vi "Try Match Response.vi"(8 "error in":errorcluster, 10 "ICAN CC Frame":refnum<class "ICAN CC Frame.lvclass">, 11 "Block Upload End Transfer in":refnum<class "Block Upload End Transfer.lvclass">) -> (0 "error out":errorcluster, 1 "SDO Result":T1={"Success"=FALSE, "SDO abort code"={"Null"=TRUE, "Value"=84082688}, "Data"={"Null"=TRUE, "Data"=[]}} {"SDO abort code"."Value" items=["Toggle bit not allowed"=84082688, "SDO protocol timed out"=84148224, "Client/server command specifier not valid or unknown"=84148225, "Invalid block size (block mode only)"=84148226, "Invalid sequence number (block mode only)"=84148227, "CRC error (block mode only)"=84148228, "Out of memory"=84148229, "Attempt to read a write only object"=100728833, "Attempt to write a read only object"=100728834, "Object does not exist in the object dictionary"=100794368, "Object cannot be mapped to the PDO"=100925505, "The number and length of the objects to be mapped would exceed PDO length"=100925506, "General parameter incompatibility reason"=100925507, "General internal incompatibility in the device"=100925511, "Access failed due to an hardware error"=101056512, "Data type does not match, length of service parameter does not match"=101122064, "Data type does not match, length of service parameter too high"=101122066, "Data type does not match, length of service parameter too low"=101122067, "Sub-index does not exist"=101253137, "Invalid value for parameter (download only)"=101253168, "Value of parameter written too high (download only)"=101253169, "Value of parameter written too low (download only)"=101253170, "Maximum value is less than minimum value"=101253174, "Resource not available: SDO connection"=101318691, "General error"=134217728, "Data cannot be transferred or stored to the application"=134217760, "Data cannot be transferred or stored to the application because of local control"=134217761, "Data cannot be transferred or stored to the application because of the present device stable"=134217762, "Object dictionary dynamic generation fails or no object dictionary is present (e.g. object dictionary is generated from file and generation fails because of an file error)"=134217763, "No data available"=134217764]; "Data"."Data" format="%02x"}, 2 "Match":bool, 3 "SDO Transfer out":refnum<class "SDO Transfer.lvclass">)   [LabVIEW 2020, in "CANopen.lvlib" / "SDO Manager.lvlib" / "Block Upload End Transfer.lvclass"]
uses:
  Block Upload End Transfer.lvclass
  HAL/Source/Interfaces/ICAN CC Frame/ICAN CC Frame.lvclass
  Block Upload End Transfer.lvclass/Block Upload End Transfer.ctl
  D:/git/CANopen-LabVIEW/source/SDO Manager/SDO Manager/SDO Transfer/SDO Transfer.lvclass
  D:/git/CANopen-LabVIEW/source/SDO Manager/SDO Manager/Block Upload End Transfer/Block Upload End Transfer.lvclass
  SDO Transfer/SDO Transfer.lvclass
  CANopen Message/CANopen Message.lvclass
  SDO Transfer/SDO abort code.ctl
  Typedefs/SDO Result.ctl
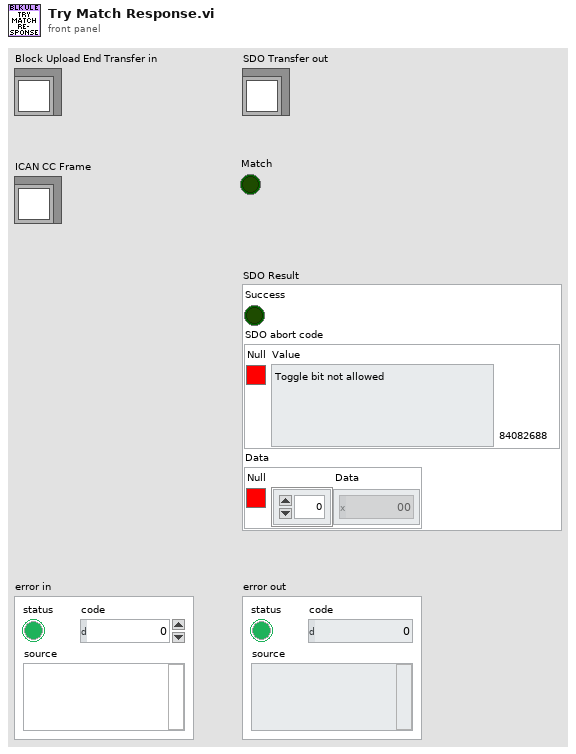
[diagram p1: front panel]
types:
  T1 = typedef "CANopen.lvlib/SDO Manager.lvlib/SDO Transfer.lvclass/SDO Result.ctl" = cluster{"Success":bool, "SDO abort code":cluster{"Null":bool, "Value":T2}, "Data":cluster{"Null":bool, "Data":u8[]}}
  T2 = typedef "CANopen.lvlib/SDO Manager.lvlib/SDO Transfer.lvclass/SDO abort code.ctl" = u32
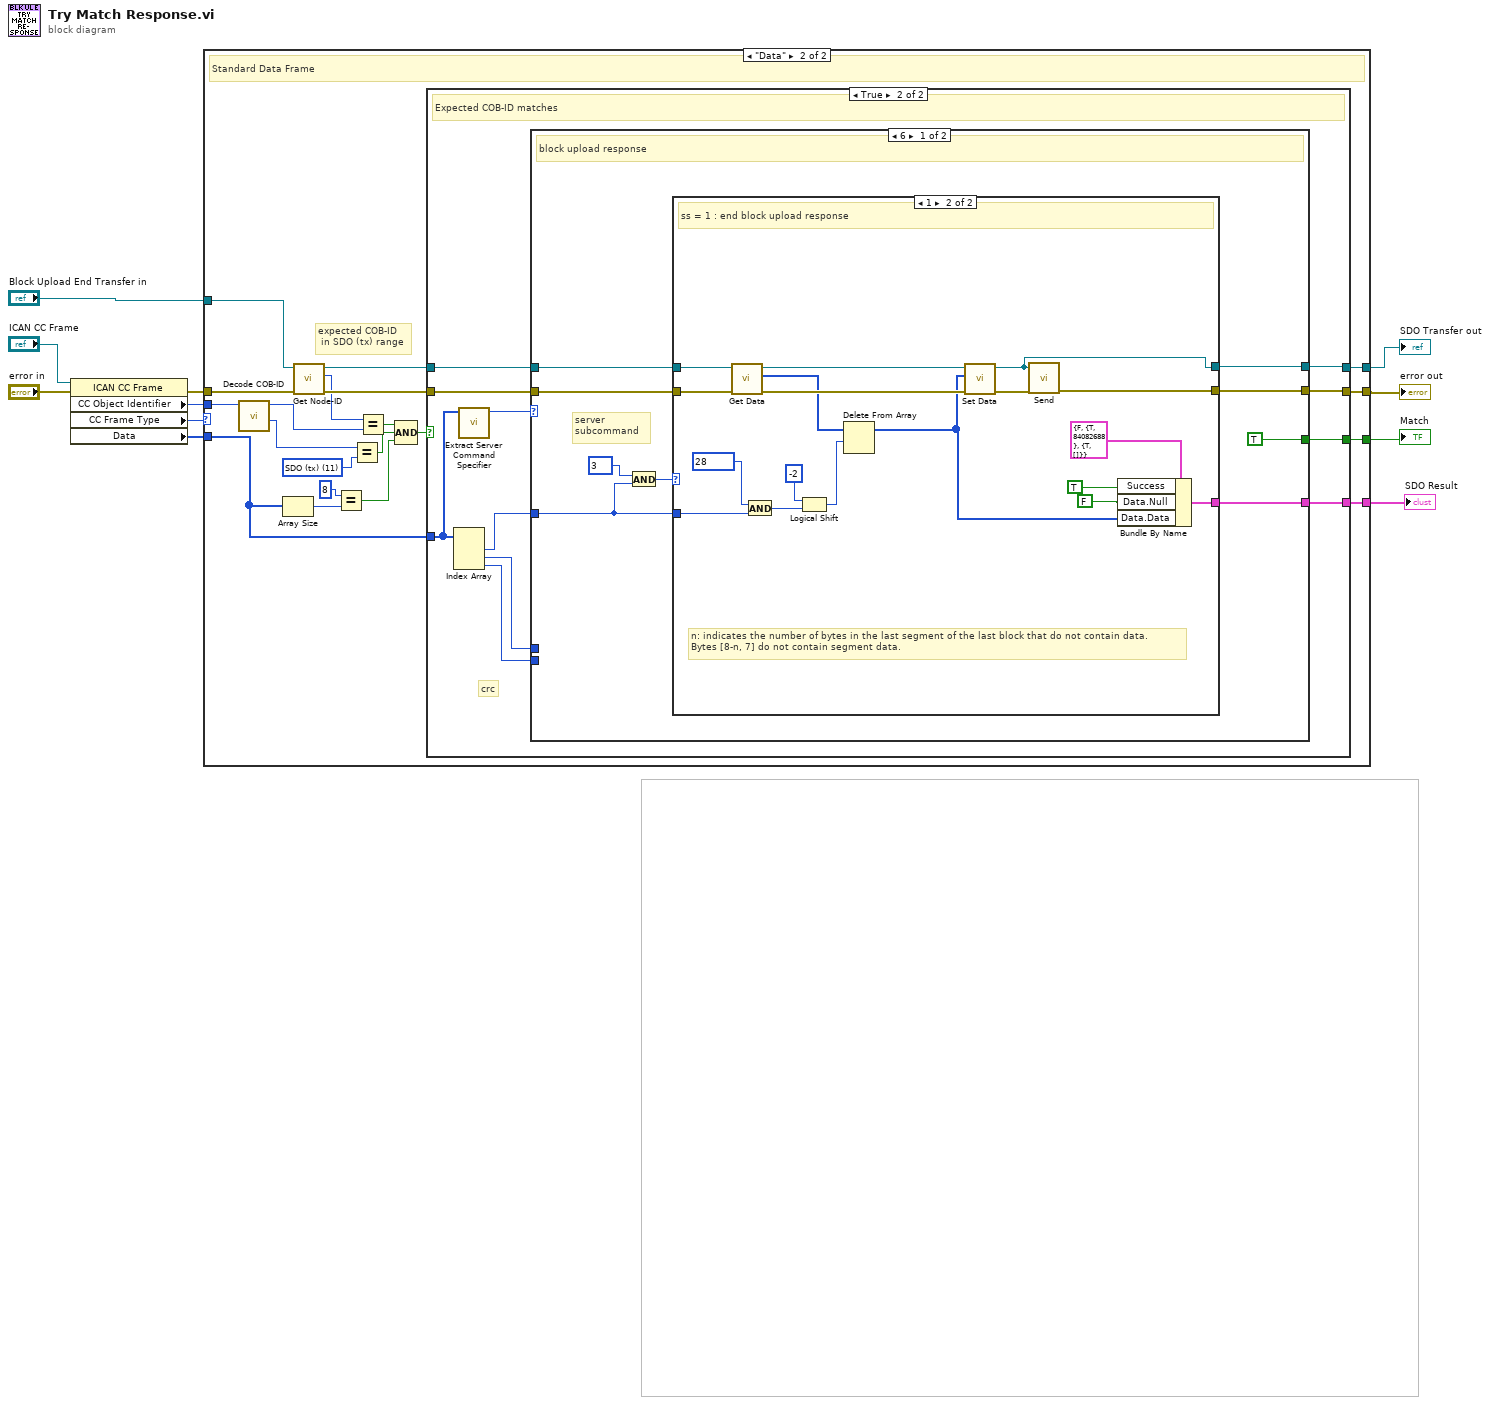
[diagram p0: block diagram]
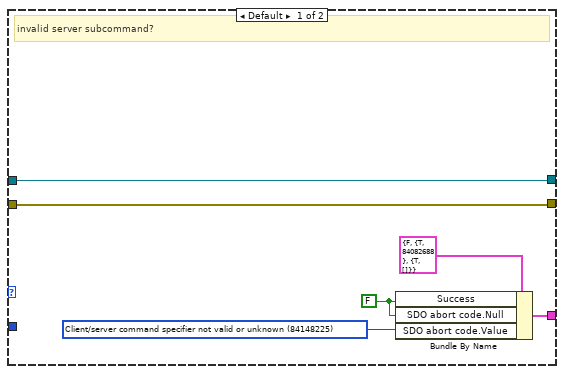
[diagram p4: hidden frame]
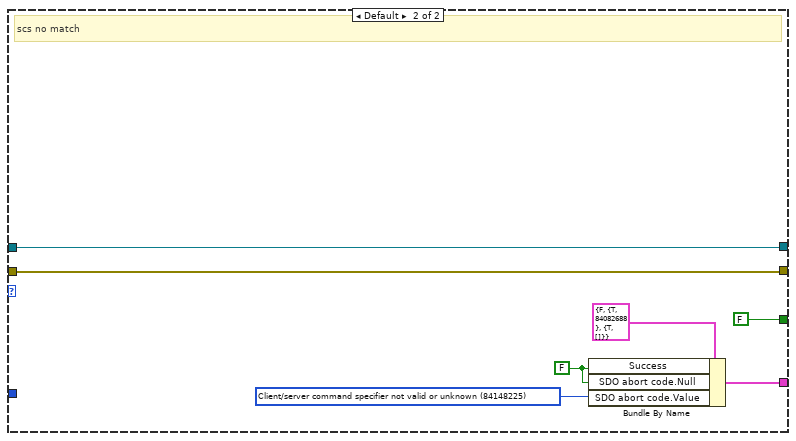
[diagram p5: hidden frame]
diagram:
  n1 = property class="ICAN CC Frame"(reference="ICAN CC Frame", error in="error in") -> (error out=w11:errorcluster, "CC Object Identifier"=w10:u32, "CC Frame Type"=w8:enum8{"Data", "Remote", "Error", "Overload"}, "Data"=w9:u8[])  [unwired: 1 out]
  n2 = case shown="\"Data\"" w8 {
    tunnel: w11 -> [w13 w33]
    tunnel: "Block Upload End Transfer in" -> [w12 w32]
    tunnel: [w12 w29] -> w5
    tunnel: [w13 w28] -> w7
    tunnel: [_ w27] -> w6
    tunnel: w10 -> [_ w26]
    tunnel: w9 -> [_ w15]
    tunnel: [_ w14] -> w1
    frame Default {
      # "Wrong Frame Type"
    }
    frame "Data" {
      w23 = u8 11 items=["NMT"=0, "EMCY/SYNC"=1, "TIME"=2, "PDO1 (tx)"=3, "PDO1 (rx)"=4, "PDO2 (tx)"=5, "PDO2 (rx)"=6, "PDO3 (tx)"=7, "PDO3 (rx)"=8, "PDO4 (tx)"=9, "PDO4 (rx)"=10, "SDO (tx)"=11, "SDO (rx)"=12, "NMT error control"=14] ("Function Code")
      # "expected COB-ID\n in SDO (tx) range"
      # "Standard Data Frame"
      n3 = call "Decode COB-ID.vi"("COD-ID"=w26) -> ("Function Code"=w22:u8, "Node-ID"=w25:u8)  [unwired: 9 in]
      n4 = Array Size(array=w15) -> (size(s)=w21:i32)
      n5 = call "Get Node-ID.vi"("error in"=w33, "SDO Transfer in"=w32) -> ("error out"=w30:errorcluster, "Node-ID"=w24:u8, "SDO Transfer out"=w31:refnum<class "Block Upload End Transfer.lvclass">)  [unwired: 7 in]
      n6 = Equal?(x=8, y=w21) -> (x = y?=w16:bool)
      n7 = Equal?(x=w22, y=w23) -> (x = y?=w17:bool)
      n8 = Equal?(x=w24, y=w25) -> (x = y?=w18:bool)
      n9 = Compound Arithmetic op=AND(w18, w17, w16) -> (w19:bool)
      n10 = case shown="True" w19 {
        tunnel: w31 -> [w35 w46]
        tunnel: w30 -> [w34 w45]
        tunnel: [w35 w41] -> w29
        tunnel: [w34 w42] -> w28
        tunnel: w15 -> [_ w38]
        tunnel: [_ w40] -> w27
        tunnel: [_ w36] -> w14
        frame False {
          # "no match"
        }
        frame True {
          # "crc"
          # "Expected COB-ID matches"
          n11 = Index Array(array=w38) -> (element #1=w39:u8, element #2=w44:u8, element #3=w43:u8)  [unwired: 3 in]
          n12 = call "Extract Server Command Specifier.vi"("Data"=w38) -> ("Server Command Specifier"=w37:u8)  [unwired: 10 in]
          n13 = case shown="6" w37 {
            tunnel: w44 -> [_ _]
            tunnel: w43 -> [_ _]
            tunnel: w46 -> [w52 w84]
            tunnel: w45 -> [w51 w86]
            tunnel: [w49 w84] -> w41
            tunnel: [w50 w86] -> w42
            tunnel: [TRUE FALSE] -> w40
            tunnel: w39 -> [w53 _]
            tunnel: [w47 w80] -> w36
            frame 6 {
              # "server\nsubcommand"
              # "block upload response"
              n14 = And(x=u8 3, y=w53) -> (x .and. y?=w54:u8)
              n15 = case shown="1" w54 {
                tunnel: w53 -> [_ w76]
                tunnel: w52 -> [w60 w74]
                tunnel: w51 -> [w61 w78]
                tunnel: [w61 w79] -> w50
                tunnel: [w60 w67] -> w49
                tunnel: [w58 w66] -> w47
                frame Default {
                  w56 = FALSE ("Success")
                  w57 = T2 84148225 items=["Toggle bit not allowed"=84082688, "SDO protocol timed out"=84148224, "Client/server command specifier not valid or unknown"=84148225, "Invalid block size (block mode only)"=84148226, "Invalid sequence number (block mode only)"=84148227, "CRC error (block mode only)"=84148228, "Out of memory"=84148229, "Attempt to read a write only object"=100728833, "Attempt to write a read only object"=100728834, "Object does not exist in the object dictionary"=100794368, "Object cannot be mapped to the PDO"=100925505, "The number and length of the objects to be mapped would exceed PDO length"=100925506, "General parameter incompatibility reason"=100925507, "General internal incompatibility in the device"=100925511, "Access failed due to an hardware error"=101056512, "Data type does not match, length of service parameter does not match"=101122064, "Data type does not match, length of service parameter too high"=101122066, "Data type does not match, length of service parameter too low"=101122067, "Sub-index does not exist"=101253137, "Invalid value for parameter (download only)"=101253168, "Value of parameter written too high (download only)"=101253169, "Value of parameter written too low (download only)"=101253170, "Maximum value is less than minimum value"=101253174, "Resource not available: SDO connection"=101318691, "General error"=134217728, "Data cannot be transferred or stored to the application"=134217760, "Data cannot be transferred or stored to the application because of local control"=134217761, "Data cannot be transferred or stored to the application because of the present device stable"=134217762, "Object dictionary dynamic generation fails or no object dictionary is present (e.g. object dictionary is generated from file and generation fails because of an file error)"=134217763, "No data available"=134217764] ("SDO abort code")
                  # "invalid server subcommand?"
                  n16 = Bundle By Name(cluster=T1 {"Success"=FALSE, "SDO abort code"={"Null"=TRUE, "Value"=84082688}, "Data"={"Null"=TRUE, "Data"=[]}} ("SDO Result"), "Success"=w56, "SDO abort code.Null"=w56, "SDO abort code.Value"=w57) -> (w58:T1)
                }
                frame 1 {
                  # "n: indicates the number of bytes in the last segment of the last block that do not contain data.\nBytes [8-n, 7] do not contain segment data."
                  # "ss = 1 : end block upload response"
                  n17 = call "Get Data.vi"("error in"=w78, "SDO Transfer in"=w74) -> ("error out"=w75:errorcluster, "Data"=w71:u8[], "SDO Transfer out"=w72:refnum<class "Block Upload End Transfer.lvclass">)  [unwired: 7 in]
                  n18 = And(x=u8 28, y=w76) -> (x .and. y?=w69:u8)
                  n19 = Logical Shift(y=i16 -2, x=w69) -> (x << y=w70:u8)
                  n20 = Delete From Array(array=w71, length=w70) -> (array with subset deleted=w62:u8[])  [unwired: 1 in, 1 out]
                  n21 = call "Set Data.vi"("error in"=w75, "Data"=w62, "SDO Transfer in"=w72) -> ("error out"=w73:errorcluster, "SDO Transfer out"=w67:refnum<class "Block Upload End Transfer.lvclass">)  [unwired: 7 in]
                  n22 = call-dynamic "Send.vi"("error in"=w73, "Block Upload End Transfer in"=w67) -> ("error out"=w79:errorcluster)  [unwired: 9 in]
                  n23 = Bundle By Name(cluster=T1 {"Success"=FALSE, "SDO abort code"={"Null"=TRUE, "Value"=84082688}, "Data"={"Null"=TRUE, "Data"=[]}} ("SDO Result"), "Success"=TRUE, "Data.Null"=FALSE, "Data.Data"=w62) -> (w66:T1)
                }
              }
            }
            frame Default {
              w81 = FALSE ("Success")
              w82 = T2 84148225 items=["Toggle bit not allowed"=84082688, "SDO protocol timed out"=84148224, "Client/server command specifier not valid or unknown"=84148225, "Invalid block size (block mode only)"=84148226, "Invalid sequence number (block mode only)"=84148227, "CRC error (block mode only)"=84148228, "Out of memory"=84148229, "Attempt to read a write only object"=100728833, "Attempt to write a read only object"=100728834, "Object does not exist in the object dictionary"=100794368, "Object cannot be mapped to the PDO"=100925505, "The number and length of the objects to be mapped would exceed PDO length"=100925506, "General parameter incompatibility reason"=100925507, "General internal incompatibility in the device"=100925511, "Access failed due to an hardware error"=101056512, "Data type does not match, length of service parameter does not match"=101122064, "Data type does not match, length of service parameter too high"=101122066, "Data type does not match, length of service parameter too low"=101122067, "Sub-index does not exist"=101253137, "Invalid value for parameter (download only)"=101253168, "Value of parameter written too high (download only)"=101253169, "Value of parameter written too low (download only)"=101253170, "Maximum value is less than minimum value"=101253174, "Resource not available: SDO connection"=101318691, "General error"=134217728, "Data cannot be transferred or stored to the application"=134217760, "Data cannot be transferred or stored to the application because of local control"=134217761, "Data cannot be transferred or stored to the application because of the present device stable"=134217762, "Object dictionary dynamic generation fails or no object dictionary is present (e.g. object dictionary is generated from file and generation fails because of an file error)"=134217763, "No data available"=134217764] ("SDO abort code")
              # "scs no match"
              n24 = Bundle By Name(cluster=T1 {"Success"=FALSE, "SDO abort code"={"Null"=TRUE, "Value"=84082688}, "Data"={"Null"=TRUE, "Data"=[]}} ("SDO Result"), "Success"=w81, "SDO abort code.Null"=w81, "SDO abort code.Value"=w82) -> (w80:T1)
            }
          }
        }
      }
    }
  }
  "SDO Transfer out" <- w5
  "error out" <- w7
  "Match" <- w6
  "SDO Result" <- w1
